vi "Get Unsupported Frequency Message.vi"(0 "Frequencies":dbl[](array[numeric]), 5 "Maximum Frequency":dbl, 7 "Minimum Frequency":dbl, 11 "error in":errorcluster, 12 "DUT Pin":string, 13 "DUT Site":i32) -> (4 "Unspported Frequency Message":string, 15 "error out":errorcluster)   [LabVIEW 2023, in "RFFixtureCharact.Public.lvlib" / "Scalar Path.lvclass"]
uses:
  Scalar Path.lvclass
  <vilib>/Utility/error.llb/Trim Whitespace One-Sided.vi
  Scalar Path.lvclass/Scalar Path.ctl
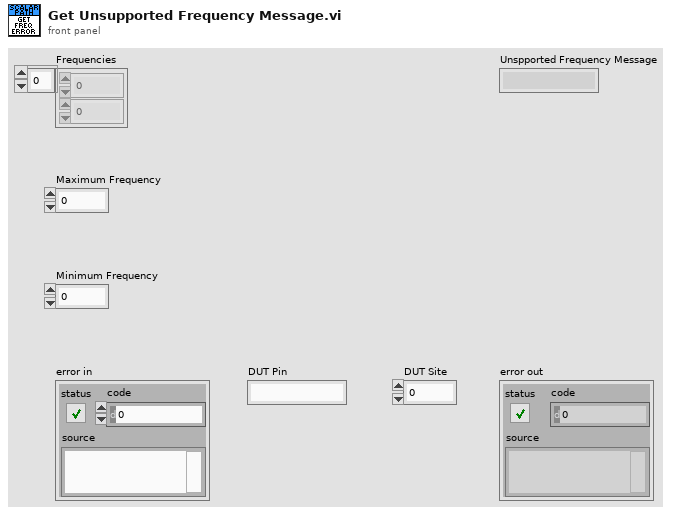
[diagram p1: front panel]
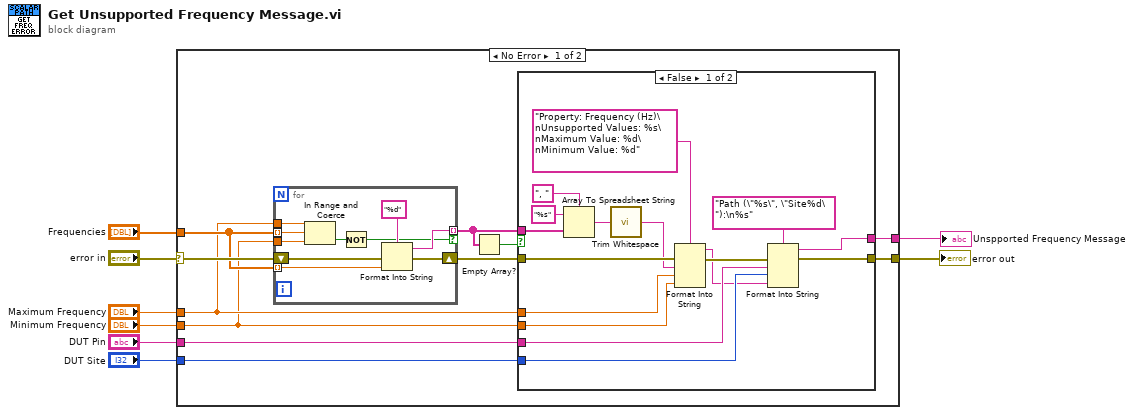
[diagram p0: block diagram]
diagram:
  n1 = case shown="No Error" "error in" {
    selector: "error in" -> [w16 w47]
    tunnel: "Frequencies" -> [w14 _]
    tunnel: "Maximum Frequency" -> [w13 _]
    tunnel: "Minimum Frequency" -> [w12 _]
    tunnel: [w9 _] -> w1
    tunnel: "DUT Pin" -> [w19 _]
    tunnel: "DUT Site" -> [w18 _]
    tunnel: [w17 w47] -> w3
    frame No Error {
      n2 = for {
        tunnel: [w29] -> w10 mode=indexing if=w20
        tunnel: w14 -> [w25] mode=indexing
        shift-right: [w26] -> w15
        shift-left: w16 -> [w27]
        tunnel: w14 -> [w24] mode=indexing
        tunnel: w13 -> [w23]
        tunnel: w12 -> [w22]
        n3 = In Range and Coerce(upper limit=w23, x=w24, lower limit=w22) -> (In Range?=w21:bool)  [unwired: 1 out]
        n4 = Not(x=w21) -> (.not. x?=w20:bool)
        n5 = Format Into String(format string="%d", error in=w27, w25) -> (resulting string=w29:string, error out=w26:errorcluster)  [unwired: 1 in]
      }
      n6 = Empty Array?(array=w10) -> (empty?=w11:bool)
      n7 = case shown="False" w11 {
        tunnel: [w30 _] -> w9
        tunnel: w19 -> [w34 _]
        tunnel: w18 -> [w35 _]
        tunnel: [w45 w46] -> w17
        tunnel: w10 -> [w42 _]
        tunnel: w15 -> [w38 w46]
        tunnel: w13 -> [w37 _]
        tunnel: w12 -> [w36 _]
        frame False {
          n8 = Array To Spreadsheet String(delimiter (Tab)=", ", array=w42, 3:"%s" ("format string")) -> (spreadsheet string=w41:string)
          n9 = call <vilib>:"Trim Whitespace.vi"("string"=w41) -> ("trimmed string"=w31:string)  [unwired: 1 in]
          n10 = Format Into String(format string="Property: Frequency (Hz)\nUnsupported Values: %s\nMaximum Value: %d\nMinimum Value: %d", error in=w38, w31, w37, w36) -> (resulting string=w33:string, error out=w39:errorcluster)  [unwired: 1 in]
          n11 = Format Into String(format string="Path (\"%s\", \"Site%d\"):\n%s", error in=w39, w34, w35, w33) -> (resulting string=w30:string, error out=w45:errorcluster)  [unwired: 1 in]
        }
        frame True {
        }
      }
    }
    frame Error {
    }
  }
  "error out" <- w3
  "Unspported Frequency Message" <- w1
